vi "Connect.vi"(0 "Embedded Exe File":path=path "Hardware Setup Files/adk.x", 5 "Hardware Setup File":path=path "Hardware Setup Files/uAutolabIII/HardwareSetup.xml", 11 "error in (no error)":errorcluster) -> (2 "Adc":refnum<k24>, 3 "Dac":refnum<k24>, 4 "Dio":refnum<k24>, 6 "Sampler":refnum<k24>, 8 "AutolabConnection":refnum<k24>, 10 "instrument":refnum<k24>, 14 "Ei":refnum<k24>, 15 "error out":errorcluster)   [LabVIEW 2011]
doc: "Connect and create an instrument. Always use Release subVI to release the instrument when stopping the application."
uses:
  C:/Program Files/Metrohm Autolab/Autolab SDK 1.10/EcoChemie.Autolab.Sdk.dll
  EcoChemie.Autolab.Sdk.dll
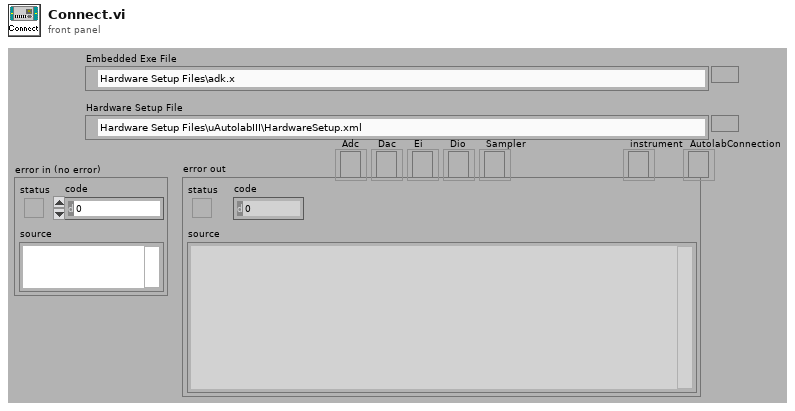
[diagram p1: front panel]
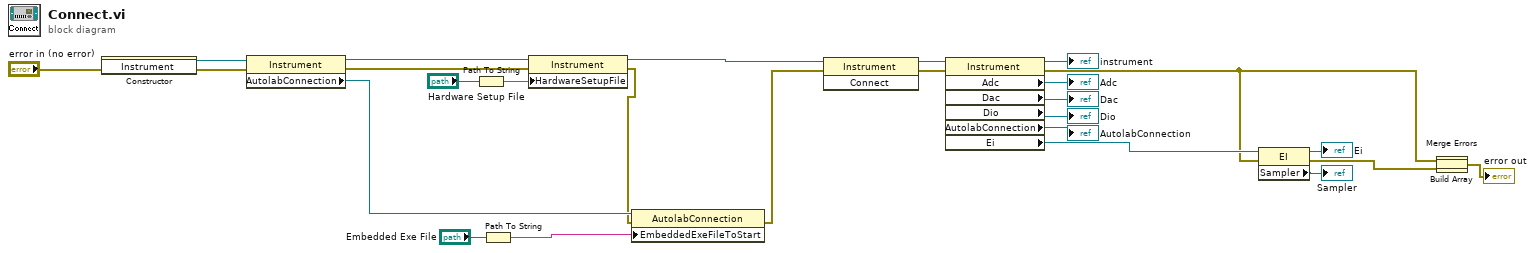
[diagram p0: block diagram]
diagram:
  n1 = constructor class="Instrument"(error in="error in (no error)") -> (reference out=w16:refnum<k24>, error out=w27:errorcluster)  [unwired: 2 in, 1 out]
  n2 = property class="Instrument"(reference=w16, error in=w27) -> (reference out=w14:refnum<k24>, error out=w13:errorcluster, "AutolabConnection"=w24:refnum<k24>)
  n3 = Path To String(path="Hardware Setup File") -> (string=w18:string)
  n4 = Path To String(path="Embedded Exe File") -> (string=w5:string)
  n5 = property class="Instrument"(reference=w14, error in=w13, "HardwareSetupFile"=w18) -> (reference out=w15:refnum<k24>, error out=w3:errorcluster)
  n6 = property class="AutolabConnection"(reference=w24, error in=w3, "EmbeddedExeFileToStart"=w5) -> (error out=w2:errorcluster)  [unwired: 1 out]
  n7 = invoke class="Instrument" method="Connect"(reference=w15, error in=w2) -> (reference out=w23:refnum<k24>, error out=w22:errorcluster)  [unwired: 1 in, 1 out]
  n8 = property class="Instrument"(reference=w23, error in=w22) -> (reference out=→"instrument":refnum<k24>, error out=w20:errorcluster, "Adc"=→"Adc":refnum<k24>, "Dac"=→"Dac":refnum<k24>, "Dio"=→"Dio":refnum<k24>, "AutolabConnection"=→"AutolabConnection":refnum<k24>, "Ei"=w21:refnum<k24>)
  n9 = property class="EI"(reference=w21, error in=w20) -> (reference out=→"Ei":refnum<k24>, error out=w19:errorcluster, "Sampler"=→"Sampler":refnum<k24>)
  n10 = Build Array(w20, w19) -> (w1:errorcluster[])
  n11 = Merge Errors(w1) -> (→"error out":errorcluster)
